vi "CheckSunk.vi"(0 "object in":refnum<class "Battleship.lvclass">, 5 "error in (no error)":errorcluster) -> (14 "object out":refnum<class "Battleship.lvclass">, 16 "Sunk?":bool, 19 "error out":errorcluster)   [LabVIEW 2015, in "Battleship.lvclass"]
uses:
  Battleship.lvclass
  Battleship.lvclass/Battleship.ctl
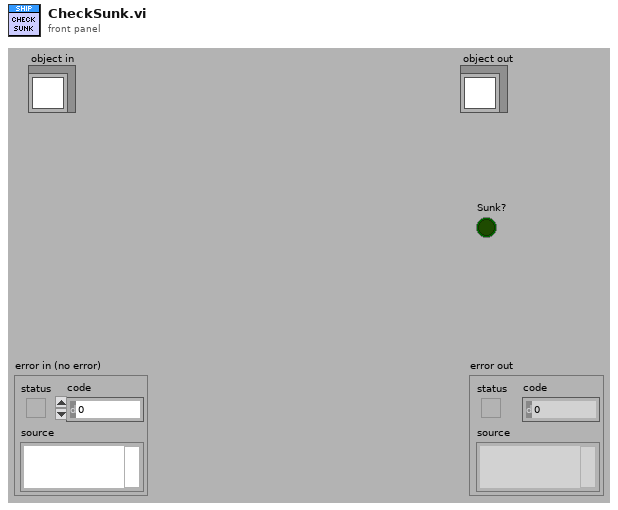
[diagram p1: front panel]
types:
  T1 = typedef "Coordinates.ctl" = cluster{"X":i32, "Y":i32}
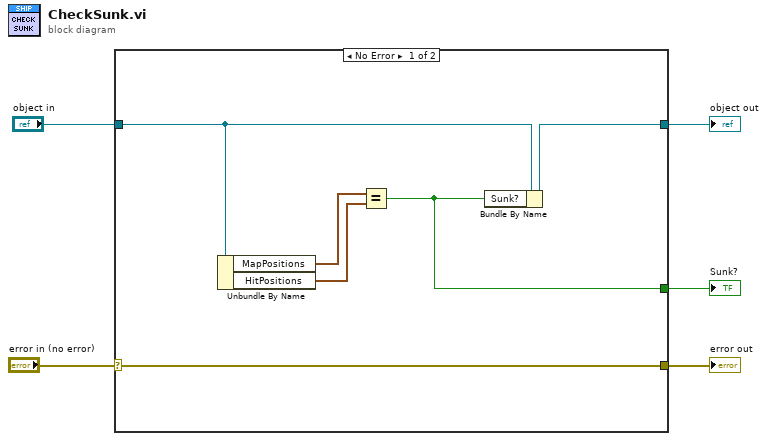
[diagram p0: block diagram]
diagram:
  n1 = case shown="No Error" "error in (no error)" {
    selector: "error in (no error)" -> [w9 w13]
    tunnel: [w9 w13] -> w4
    tunnel: [w11 w12] -> w2
    tunnel: "object in" -> [w10 w12]
    tunnel: [w8 _] -> w1
    frame No Error {
      n2 = Unbundle By Name(w10) -> ("MapPositions"=w7:T1[], "HitPositions"=w6:T1[])
      n3 = Equal?(x=w7, y=w6) -> (x = y?=w8:bool)
      n4 = Bundle By Name(cluster=w10, "Sunk?"=w8) -> (w11:refnum<class "Battleship.lvclass">)
    }
    frame Error {
    }
  }
  "error out" <- w4
  "object out" <- w2
  "Sunk?" <- w1
